vi "GetDLLVersion.vi"(6 "error in":errorcluster) -> (0 "error out":errorcluster, 2 "DLL Version":string)   [LabVIEW 2018]
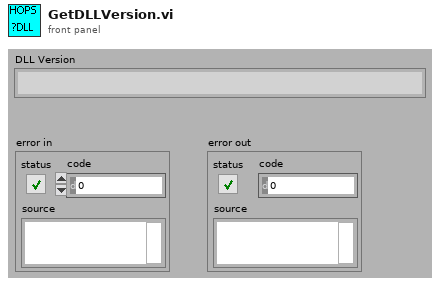
[diagram p1: front panel]
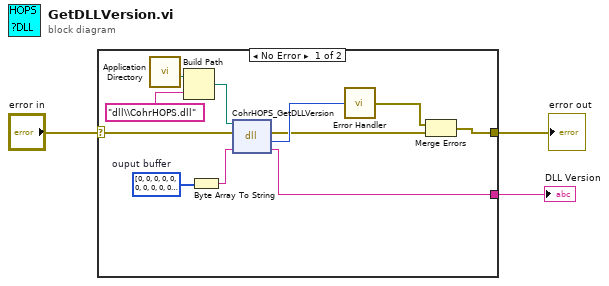
[diagram p0: block diagram]
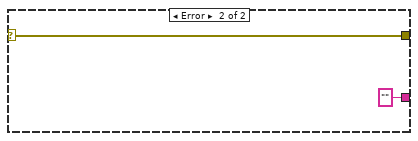
[diagram p2: hidden frame]
diagram:
  n1 = case shown="No Error" "error in" {
    selector: "error in" -> [w12 w15]
    tunnel: [w13 ""] -> w3
    tunnel: [w11 w15] -> w2
    frame No Error {
      w8 = u8[] [0, 0, 0, 0, 0, 0, 0, 0, 0, 0, 0, 0, 0, 0, 0, 0, 0, 0, 0, 0, 0, 0, 0, 0, 0, 0, 0, 0, 0, 0, 0, 0, 0, 0, 0, 0, 0, 0, 0, 0, 0, 0, 0, 0, 0, 0, 0, 0, 0, 0, 0, 0, 0, 0, 0, 0, 0, 0, 0, 0, 0, 0, 0, 0, 0, 0, 0, 0, 0, 0, 0, 0, 0, 0, 0, 0, 0, 0, 0, 0, 0, 0, 0, 0, 0, 0, 0, 0, 0, 0, 0, 0, 0, 0, 0, 0, 0, 0, 0, 0, 1]  # ouput buffer
      n2 = call <vilib>:"Application Directory.vi"() -> ("Application Directory"=w6:path)
      n3 = Build Path(base path=w6, name or relative path="dll\\CohrHOPS.dll") -> (appended path=w4:path)
      n4 = Byte Array To String(unsigned byte array=w8) -> (string=w7:string)
      n5 = dll-call lib="?" fn="CohrHOPS_GetDLLVersion"(path in=w4, error in=w12, w7) -> (error out=w9:errorcluster, "return type"=w14:i32, w13:string)  [unwired: 1 in, 1 out]
      n6 = call "Error Handler.vi"("Return Value"=w14) -> ("error out"=w10:errorcluster)
      n7 = Merge Errors(w10, w9) -> (w11:errorcluster)
    }
    frame Error {
    }
  }
  "DLL Version" <- w3
  "error out" <- w2
